vi "states.vi"(0 "keithley":T1, 4 "LVTTiSEH":T1, 6 "inverter":T1, 8 "Chiller":T1, 9 "DeltaPS":T1, 10 "Array":string[](array[string]), 11 "String":string) -> (3 "String 2":string)   [LabVIEW 2019]
uses:
  Keithley/Keithley 24XX/Keithley 24XX.lvlib
panel:
  in  "stop reading script":bool
  out "From Linux Box":string
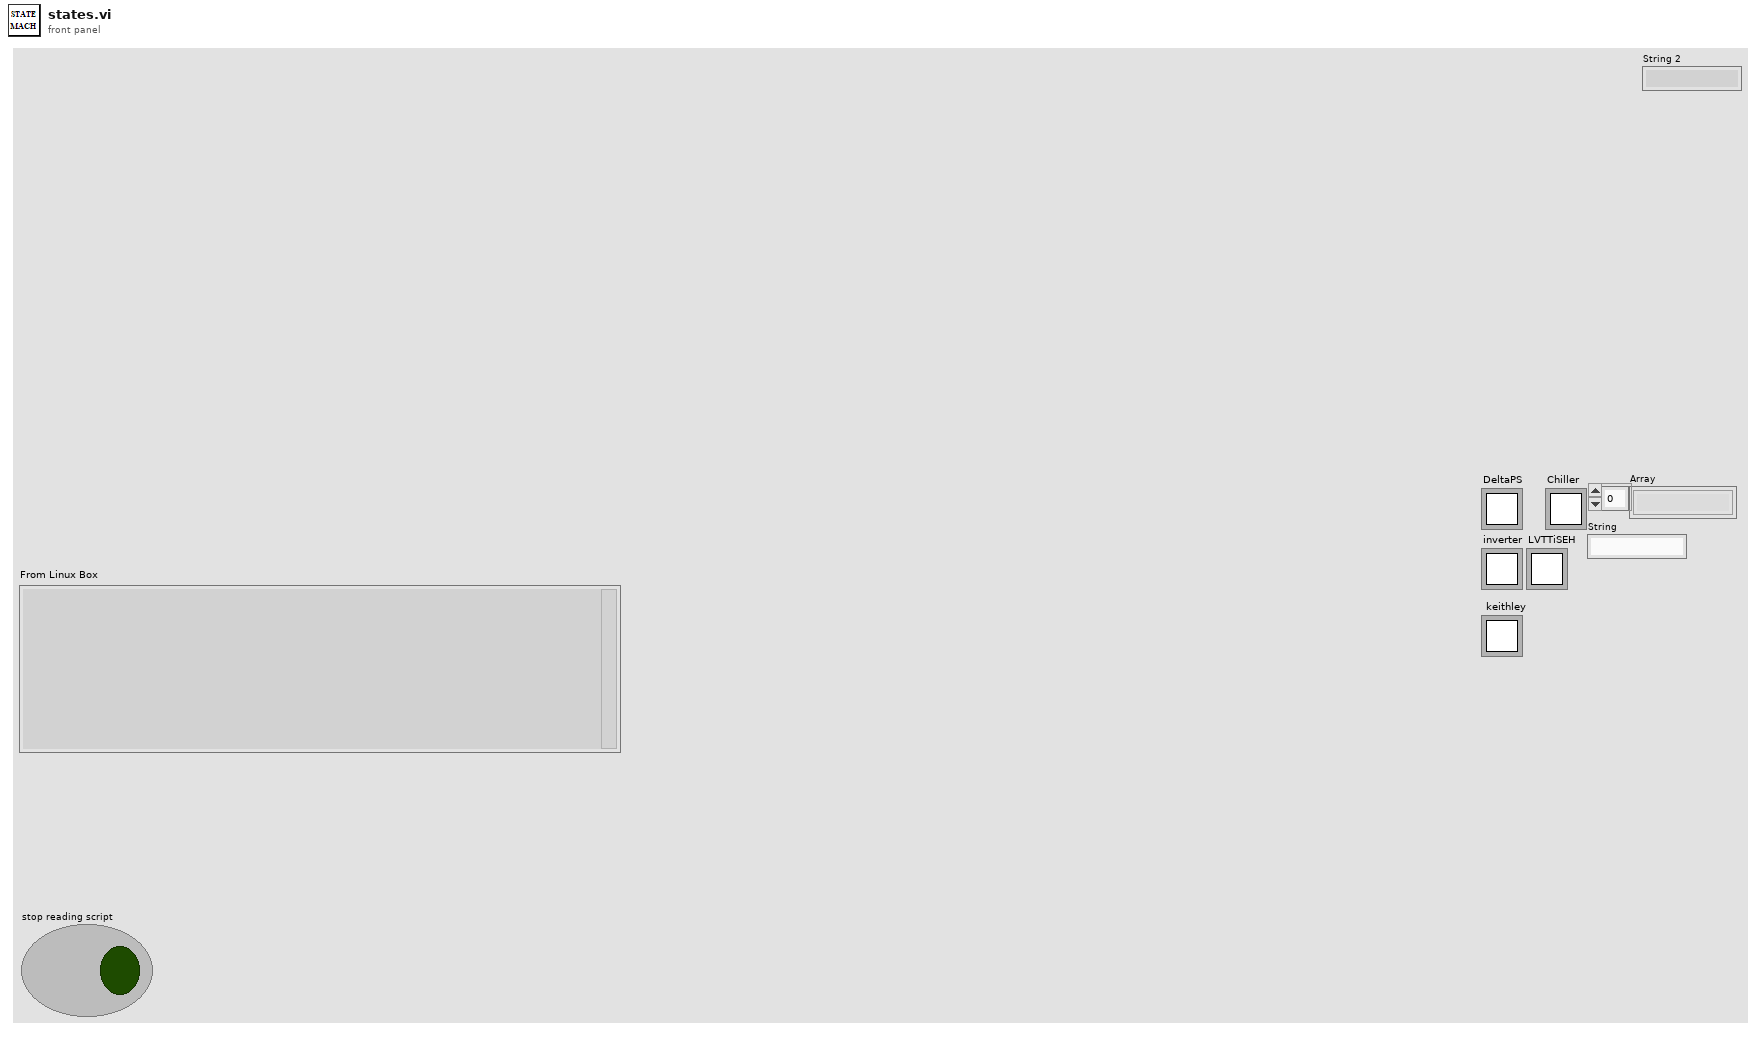
[diagram p1: front panel]
types:
  T1 = typedef "Semaphore RefNum" = refnum<k1>
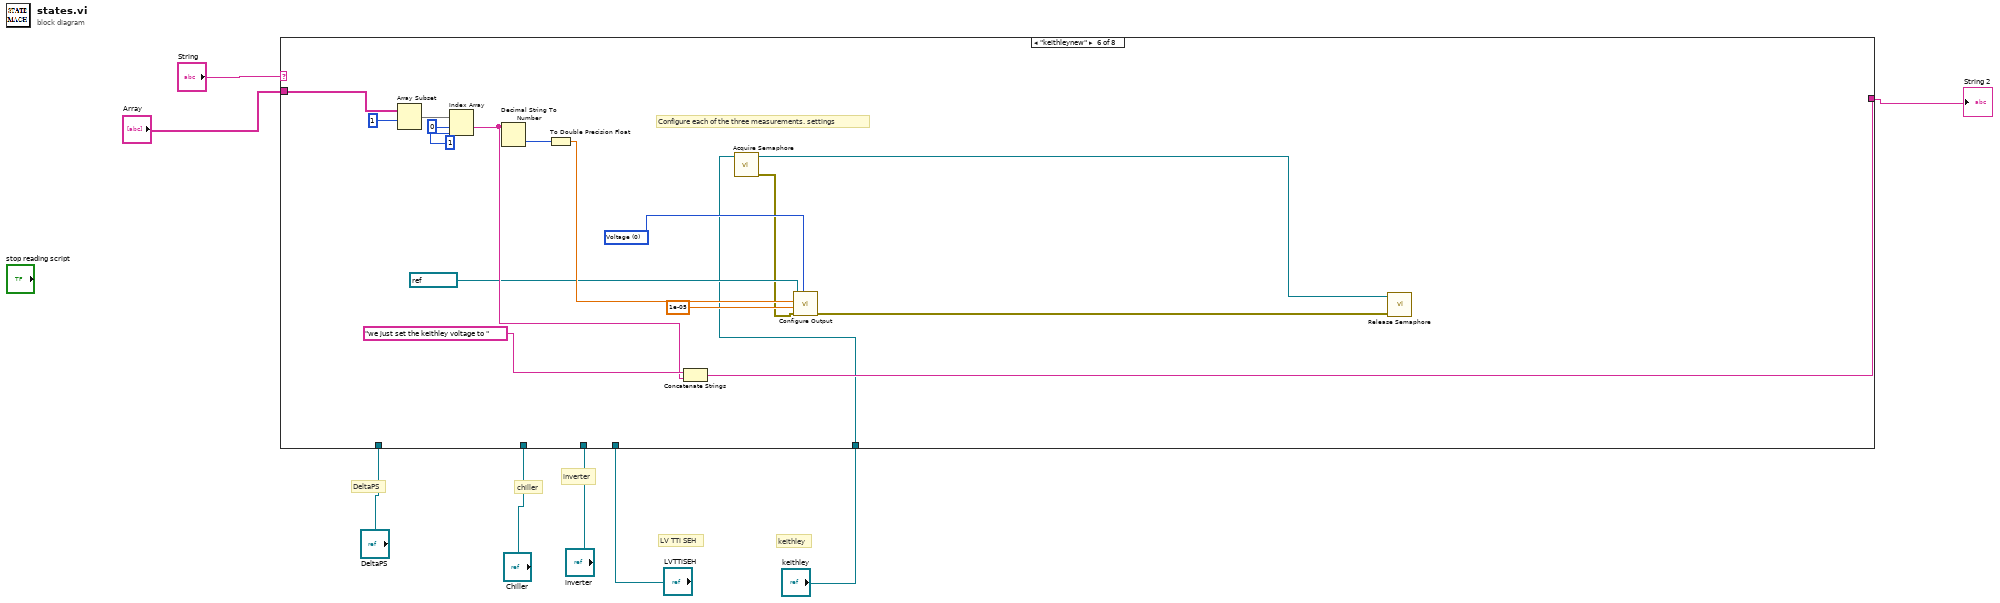
[diagram p0: block diagram]
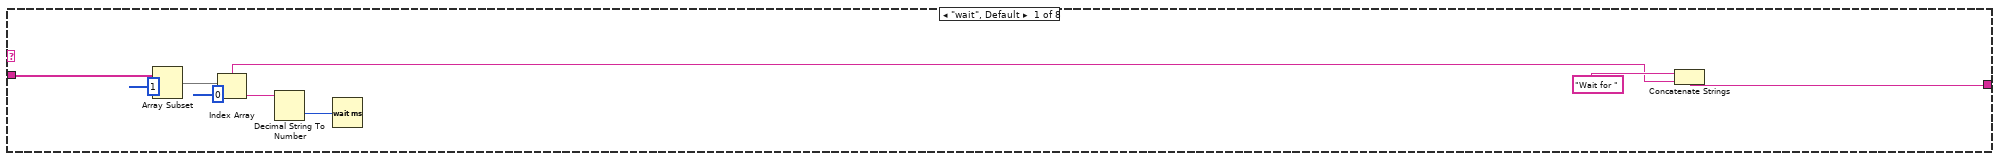
[diagram p2: hidden frame]
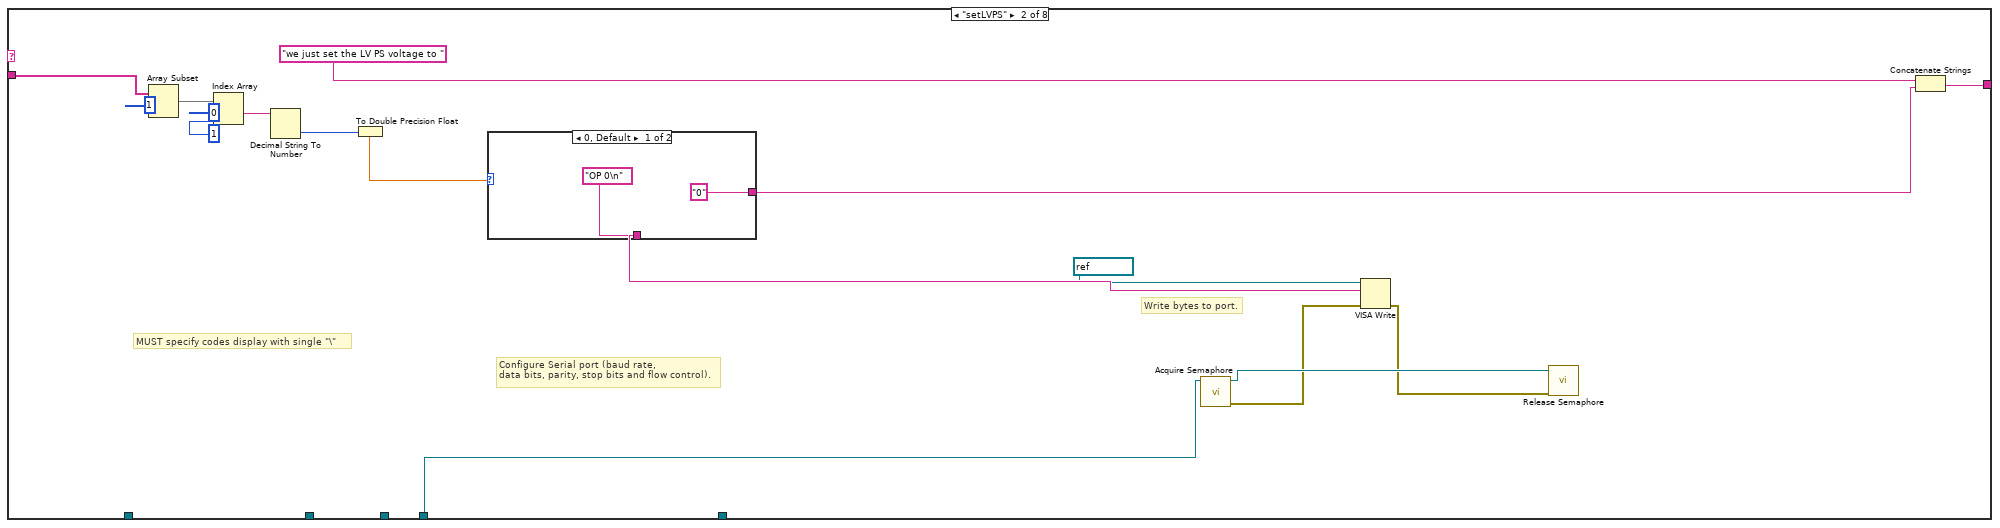
[diagram p3: hidden frame]
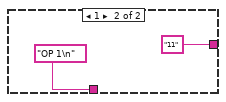
[diagram p4: hidden frame]
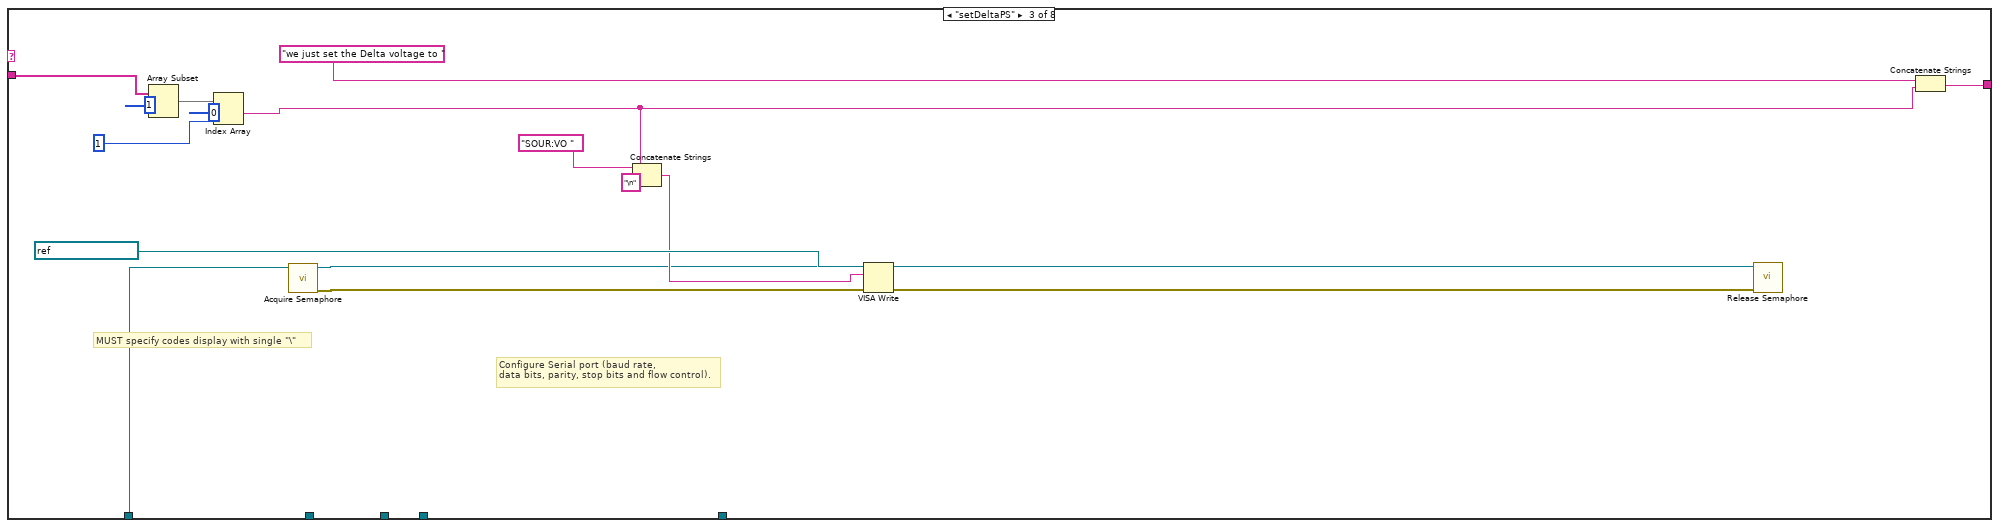
[diagram p5: hidden frame]
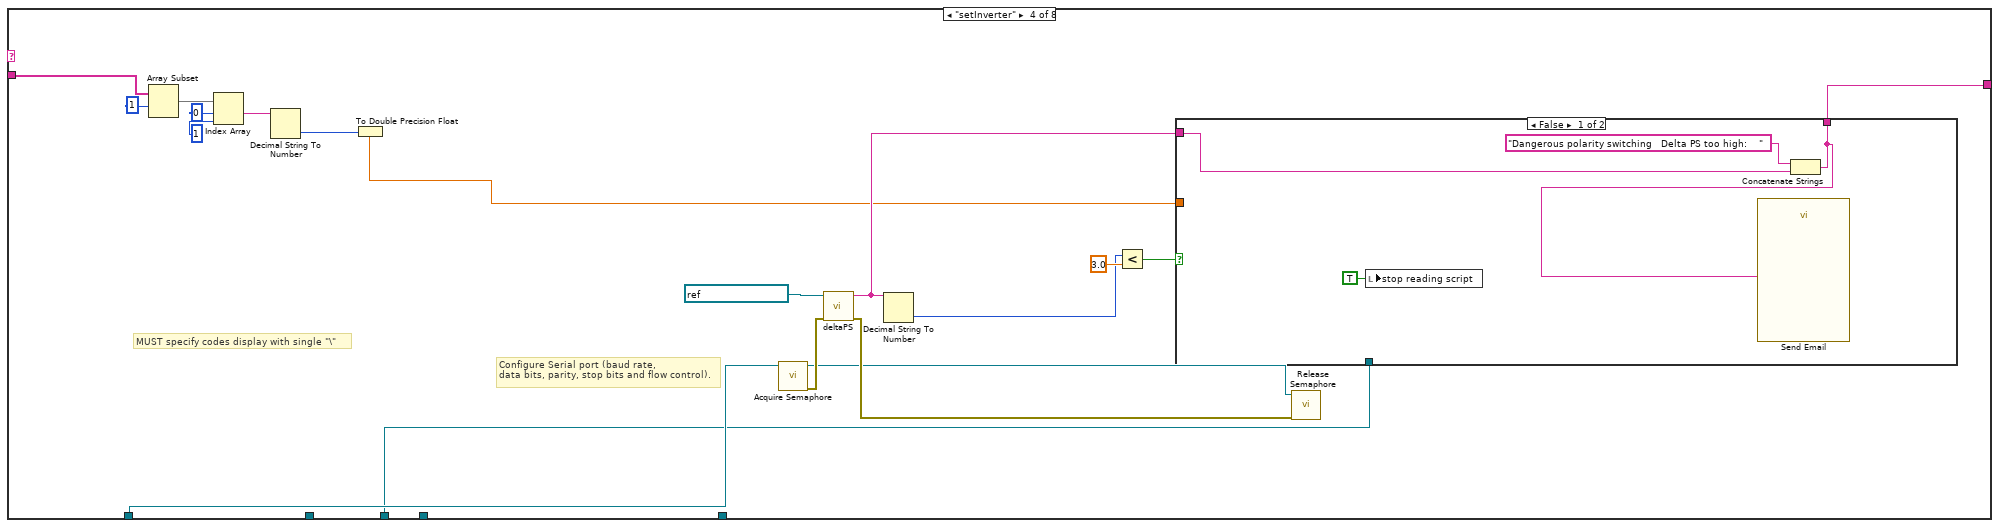
[diagram p6: hidden frame]
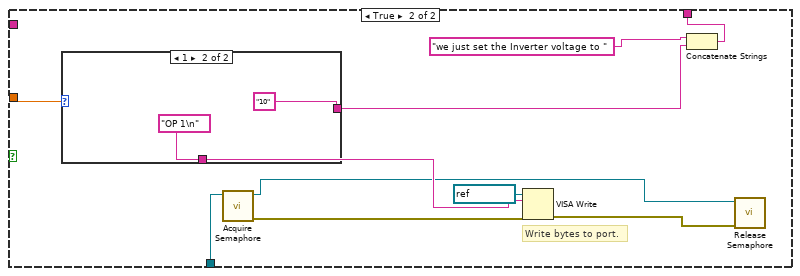
[diagram p7: hidden frame]
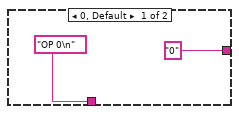
[diagram p8: hidden frame]
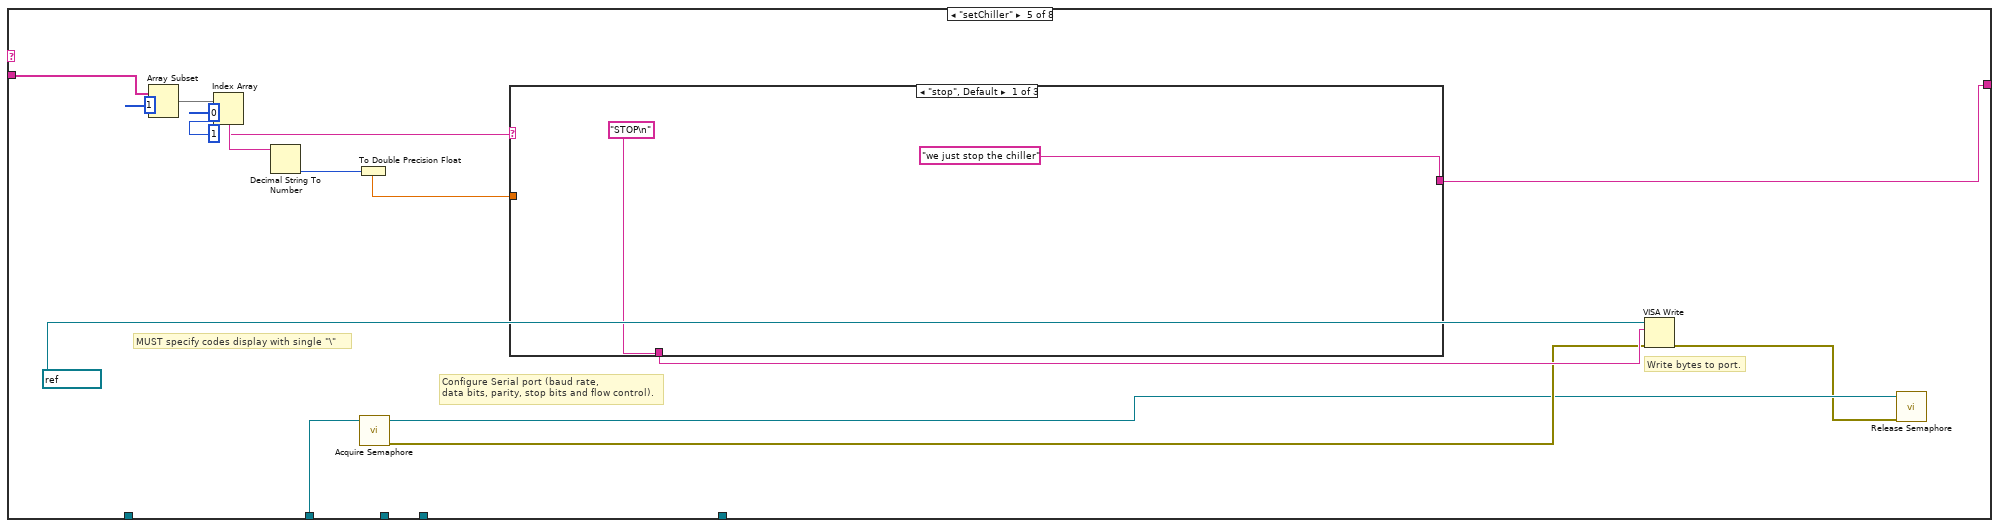
[diagram p9: hidden frame]
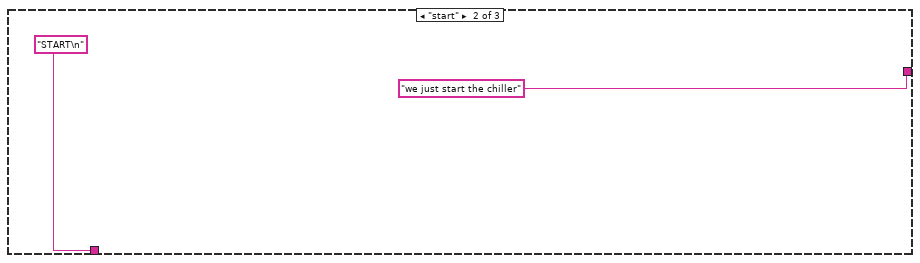
[diagram p10: hidden frame]
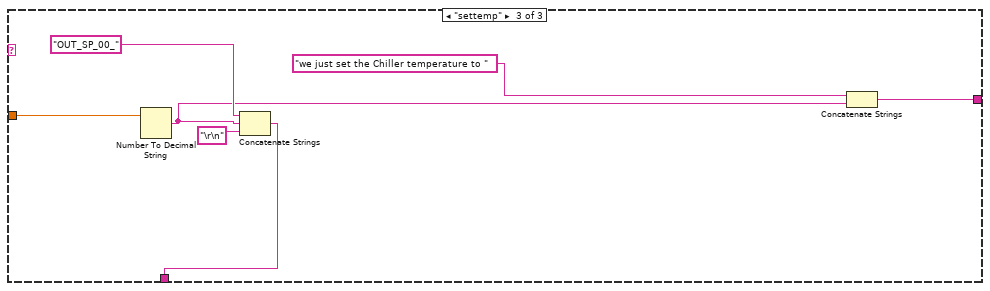
[diagram p11: hidden frame]
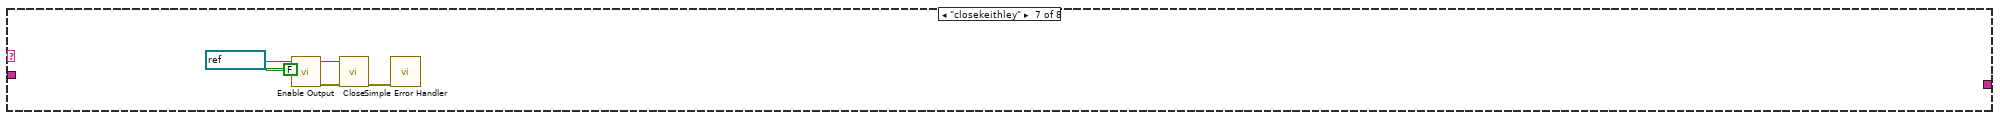
[diagram p12: hidden frame]
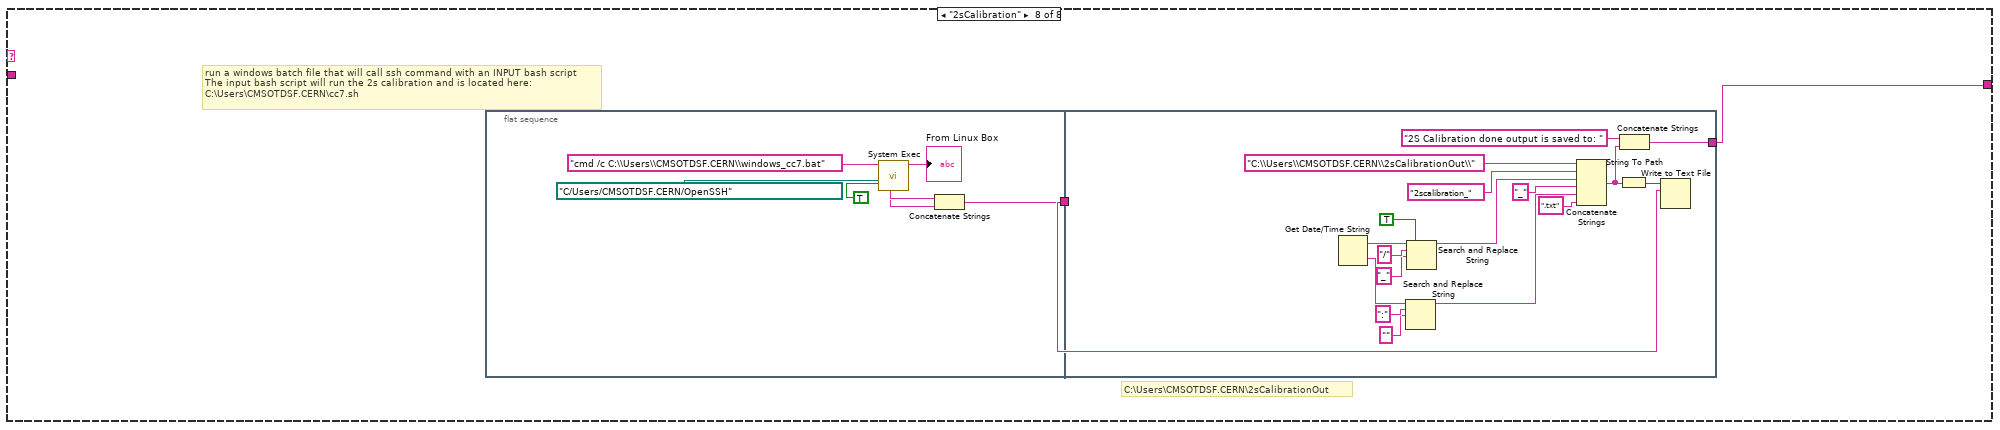
[diagram p13: hidden frame]
diagram:
  # "keithley"
  # "LV TTi SEH"
  # "inverter"
  # "chiller"
  # "DeltaPS"
  n1 = case shown="\"keithleynew\"" "String" {
    tunnel: "Array" -> [w16 w28 w49 w67 w102 w131 _ _]
    tunnel: [w9 w25 w47 w59 w95 w127 _ w140] -> w2
    tunnel: "DeltaPS" -> [_ _ w41 w58 _ _ _ _]
    tunnel: "Chiller" -> [_ _ _ _ w94 _ _ _]
    tunnel: "inverter" -> [_ _ _ w54 _ _ _ _]
    tunnel: "LVTTiSEH" -> [_ w17 _ _ _ _ _ _]
    tunnel: "keithley" -> [_ _ _ _ _ w119 _ _]
    frame "wait", Default {
      n2 = Array Subset(array=w16, index=1) -> (w14:string[])  [unwired: 1 in]
      n3 = Index Array(array=w14, index=0) -> (element=w10:string)
      n4 = Decimal String To Number(string=w10) -> (number=w12:i32)  [unwired: 2 in, 1 out]
      n5 = Wait (ms)(milliseconds to wait=w12) -> ()  [unwired: 1 out]
      n6 = Concatenate Strings("Wait for ", w10) -> (w9:string)
    }
    frame "setLVPS" {
      # "Write bytes to port."
      # "MUST specify codes display with single \"\\\""
      # "Configure Serial port (baud rate,\ndata bits, parity, stop bits and flow control)."
      n7 = Array Subset(array=w28, index=1) -> (w33:string[])  [unwired: 1 in]
      n8 = Index Array(array=w33, index #1=0 ("index"), index #2=1 ("index")) -> (element #1=w30:string)  [unwired: 1 out]
      n9 = Decimal String To Number(string=w30) -> (number=w27:i32)  [unwired: 2 in, 1 out]
      n10 = To Double Precision Float(number=w27) -> (double precision float=w24:dbl)
      n11 = case shown="0, Default" w24 {
        tunnel: ["OP 0\n" ("Combo Box 4") "OP 1\n" ("Combo Box 4")] -> w23
        tunnel: ["0" ("Combo Box 4") "11" ("Combo Box 4")] -> w21
        frame 0, Default {
        }
        frame 1 {
        }
      }
      n12 = call <vilib>:"Acquire Semaphore.vi"("semaphore"=w17) -> ("error out"=w19:errorcluster, "semaphore out"=w20:T1)  [unwired: 4 in, 1 out]
      n13 = VISA Write(VISA resource name=refnum<visa-resource-name> "COM5", write buffer=w23, error in (no error)=w19) -> (error out=w18:errorcluster)  [unwired: 2 out]
      n14 = call <vilib>:"Release Semaphore.vi"("error in (no error)"=w18, "semaphore"=w20) -> ()  [unwired: 4 in, 2 out]
      n15 = Concatenate Strings("we just set the LV PS voltage to ", w21) -> (w25:string)
    }
    frame "setDeltaPS" {
      # "MUST specify codes display with single \"\\\""
      # "Configure Serial port (baud rate,\ndata bits, parity, stop bits and flow control)."
      n16 = Array Subset(array=w49, index=1) -> (w53:string[])  [unwired: 1 in]
      n17 = Index Array(array=w53, index #1=0 ("index"), index #2=1 ("index")) -> (element #1=w42:string)  [unwired: 1 out]
      n18 = call <vilib>:"Acquire Semaphore.vi"("semaphore"=w41) -> ("error out"=w40:errorcluster, "semaphore out"=w38:T1)  [unwired: 4 in, 1 out]
      n19 = Concatenate Strings("SOUR:VO " ("format string"), w42, "\n" ("string")) -> (w44:string)
      n20 = VISA Write(VISA resource name=refnum<visa-resource-name> "GPIB0::8::INSTR", write buffer=w44, error in (no error)=w40) -> (error out=w39:errorcluster)  [unwired: 2 out]
      n21 = call <vilib>:"Release Semaphore.vi"("error in (no error)"=w39, "semaphore"=w38) -> ()  [unwired: 4 in, 2 out]
      n22 = Concatenate Strings("we just set the Delta voltage to ", w42) -> (w47:string)
    }
    frame "setInverter" {
      # "MUST specify codes display with single \"\\\""
      # "Configure Serial port (baud rate,\ndata bits, parity, stop bits and flow control)."
      n23 = Array Subset(array=w67, index=1) -> (w72:string[])  [unwired: 1 in]
      n24 = Index Array(array=w72, index #1=0 ("index"), index #2=1 ("index")) -> (element #1=w69:string)  [unwired: 1 out]
      n25 = Decimal String To Number(string=w69) -> (number=w66:i32)  [unwired: 2 in, 1 out]
      n26 = To Double Precision Float(number=w66) -> (double precision float=w60:dbl)
      n27 = call <vilib>:"Acquire Semaphore.vi"("semaphore"=w58) -> ("error out"=w57:errorcluster, "semaphore out"=w55:T1)  [unwired: 4 in, 1 out]
      n28 = call "deltaPS.vi"("error in (no error)"=w57, "VISA Refnum in"=refnum<visa-resource-name> "GPIB0::8::INSTR" ("VISA resource name")) -> ("error out"=w56:errorcluster, "DeltaPS"=w61:string)  [unwired: 8 in]
      n29 = Decimal String To Number(string=w61) -> (number=w62:i32)  [unwired: 2 in, 1 out]
      n30 = Less?(x=w62, y=3.0) -> (x < y?=w64:bool)
      n31 = case shown="False" w64 {
        tunnel: w60 -> [_ w84]
        tunnel: w61 -> [w75 _]
        tunnel: [w74 w81] -> w59
        tunnel: w54 -> [_ w77]
        frame False {
          n32 = local write "stop reading script"(TRUE ("stop reading script")) -> ()
          n33 = Concatenate Strings("Dangerous polarity switching   Delta PS too high:    ", w75) -> (w74:string)
          n34 = call "Send Email"("Message"=w74) -> ()  [unwired: 10 in, 1 out]
        }
        frame True {
          # "Write bytes to port."
          n35 = case shown="1" w84 {
            tunnel: ["OP 0\n" ("Combo Box 4") "OP 1\n" ("Combo Box 4")] -> w86
            tunnel: ["0" ("Combo Box 4") "10" ("Combo Box 4")] -> w82
            frame 0, Default {
            }
            frame 1 {
            }
          }
          n36 = call <vilib>:"Acquire Semaphore.vi"("semaphore"=w77) -> ("error out"=w80:errorcluster, "semaphore out"=w78:T1)  [unwired: 4 in, 1 out]
          n37 = VISA Write(VISA resource name=refnum<visa-resource-name> "COM4", write buffer=w86, error in (no error)=w80) -> (error out=w79:errorcluster)  [unwired: 2 out]
          n38 = Concatenate Strings("we just set the Inverter voltage to ", w82) -> (w81:string)
          n39 = call <vilib>:"Release Semaphore.vi"("error in (no error)"=w79, "semaphore"=w78) -> ()  [unwired: 4 in, 2 out]
        }
      }
      n40 = call <vilib>:"Release Semaphore.vi"("error in (no error)"=w56, "semaphore"=w55) -> ()  [unwired: 4 in, 2 out]
    }
    frame "setChiller" {
      # "Write bytes to port."
      # "MUST specify codes display with single \"\\\""
      # "Configure Serial port (baud rate,\ndata bits, parity, stop bits and flow control)."
      n41 = Array Subset(array=w102, index=1) -> (w106:string[])  [unwired: 1 in]
      n42 = Index Array(array=w106, index #1=0 ("index"), index #2=1 ("index")) -> (element #1=w97:string, element #2=w99:string)
      n43 = Decimal String To Number(string=w99) -> (number=w98:i32)  [unwired: 2 in, 1 out]
      n44 = To Double Precision Float(number=w98) -> (double precision float=w96:dbl)
      n45 = call <vilib>:"Acquire Semaphore.vi"("semaphore"=w94) -> ("error out"=w93:errorcluster, "semaphore out"=w92:T1)  [unwired: 4 in, 1 out]
      n46 = case shown="\"stop\", Default" w97 {
        tunnel: ["STOP\n" ("Combo Box 4") "START\n" ("Combo Box 4") w115] -> w101
        tunnel: w96 -> [_ _ w114]
        tunnel: ["we just stop the chiller" "we just start the chiller" w111] -> w95
        frame "stop", Default {
        }
        frame "start" {
        }
        frame "settemp" {
          n47 = Number To Decimal String(number=w114) -> (decimal integer string=w113:string)  [unwired: 1 in]
          n48 = Concatenate Strings("OUT_SP_00_" ("Combo Box 4"), w113, "\r\n" ("string")) -> (w115:string)
          n49 = Concatenate Strings("we just set the Chiller temperature to ", w113) -> (w111:string)
        }
      }
      n50 = VISA Write(VISA resource name=refnum<visa-resource-name> "COM6", write buffer=w101, error in (no error)=w93) -> (error out=w91:errorcluster)  [unwired: 2 out]
      n51 = call <vilib>:"Release Semaphore.vi"("error in (no error)"=w91, "semaphore"=w92) -> ()  [unwired: 4 in, 2 out]
    }
    frame "keithleynew" {
      w122 = u16 0 items=["Voltage", "Current"] ("Source Mode  (0: Voltage)")
      # "Configure each of the three measurements. settings"
      n52 = Array Subset(array=w131, index=1) -> (w134:string[])  [unwired: 1 in]
      n53 = Index Array(array=w134, index #1=0 ("index"), index #2=1 ("index")) -> (element #1=w128:string)  [unwired: 1 out]
      n54 = Decimal String To Number(string=w128) -> (number=w130:i32)  [unwired: 2 in, 1 out]
      n55 = To Double Precision Float(number=w130) -> (double precision float=w125:dbl)
      n56 = Concatenate Strings("we just set the keithley voltage to ", w128) -> (w127:string)
      n57 = call <vilib>:"Acquire Semaphore.vi"("semaphore"=w119) -> ("error out"=w120:errorcluster, "semaphore out"=w121:T1)  [unwired: 4 in, 1 out]
      n58 = call "Configure Output.vi"("Source Mode  (0: Voltage)"=w122, "error in (no error)"=w120, "Compliance  Level (0.1)"=1e-05, "Output Level (0)"=w125, "VISA resource name"=refnum<visa-resource-name> "COM1") -> ("error out"=w118:errorcluster)  [unwired: 5 in, 1 out]
      n59 = call <vilib>:"Release Semaphore.vi"("error in (no error)"=w118, "semaphore"=w121) -> ()  [unwired: 4 in, 2 out]
    }
    frame "closekeithley" {
      n60 = call "Enable Output.vi"("Enable Output (T: Enable)"=FALSE, "VISA resource name"=refnum<visa-resource-name> "COM1") -> ("error out"=w136:errorcluster, "VISA resource name out"=w137:refnum<visa-resource-name>)  [unwired: 8 in]
      n61 = call "Close.vi"("error in (no error)"=w136, "VISA resource name"=w137) -> ("error out"=w139:errorcluster)  [unwired: 9 in]
      n62 = call <vilib>:"Simple Error Handler.vi"("error in (no error)"=w139) -> ()  [unwired: 4 in, 5 out]
    }
    frame "2sCalibration" {
      # "C:\\Users\\CMSOTDSF.CERN\\2sCalibrationOut"
      # "run a windows batch file that will call ssh command with an INPUT bash script\nThe input bash script will run the 2s calibration and is located here:\nC:\\Users\\CMSOTDSF.CERN\\cc7.sh"
      n63 = flat-sequence {
        tunnel: [w143] -> w141
        tunnel: w141 -> [w149]
        tunnel: [w148] -> w140
        frame #0 {
          n64 = call <vilib>:"System Exec.vi"("run minimized? (F)"=TRUE, "working directory"=path "C:/Users/CMSOTDSF.CERN/OpenSSH", "command line"="cmd /c C:\\Users\\CMSOTDSF.CERN\\windows_cc7.bat") -> ("standard error"=w144:string, "standard output"=w145:string)  [unwired: 5 in, 2 out]
          "From Linux Box" <- w145
          n65 = Concatenate Strings(w145, w144) -> (w143:string)
        }
        frame #1 {
          n66 = Get Date/Time String() -> (date string=w160:string, time string=w162:string)  [unwired: 3 in]
          n67 = Search and Replace String(input string=w162, search string=":", replace string="" ("replace string (\"\")")) -> (result string=w163:string)  [unwired: 5 in, 3 out]
          n68 = Search and Replace String(replace all?=TRUE ("replace all? (F)"), input string=w160, search string="/", replace string="_" ("replace string (\"\")")) -> (result string=w161:string)  [unwired: 4 in, 3 out]
          n69 = Concatenate Strings("C:\\Users\\CMSOTDSF.CERN\\2sCalibrationOut\\" ("string"), "2scalibration_" ("string"), w161, "_" ("string"), w163, ".txt" ("string")) -> (w164:string)
          n70 = String To Path(string=w164) -> (path=w165:path)
          n71 = Concatenate Strings("2S Calibration done output is saved to: ", w164) -> (w148:string)
          n72 = Write to Text File(file (use dialog)=w165, text=w149) -> ()  [unwired: 2 in, 3 out]
        }
      }
    }
  }
  "String 2" <- w2
